vi "GetCurrentState.vi"(1 "State Array In":string[](array[string])) -> (10 "Current State":string, 15 "State Array Out":string[](array[string]))   [LabVIEW 2018]
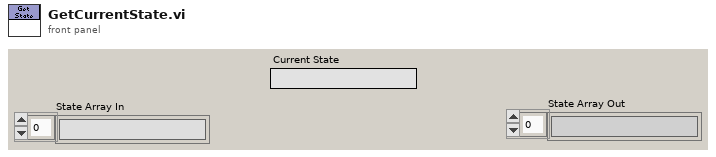
[diagram p1: front panel]
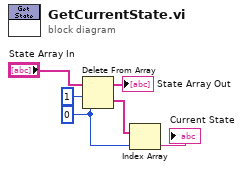
[diagram p0: block diagram]
diagram:
  w5 = 0 ("index")
  n1 = Delete From Array(array="State Array In", length=1, index=w5) -> (deleted portion=w4:string[], array with subset deleted=→"State Array Out":string[])
  n2 = Index Array(array=w4, index=w5) -> (element=→"Current State":string)
